vi "Validate Routing Channel.vi"(8 "error in (no error)":errorcluster, 11 "JSON RCT":refnum<class "JSON Routing Channel Template.lvclass">) -> (0 "error out":errorcluster, 3 "JSON RCT":refnum<class "JSON Routing Channel Template.lvclass">)   [LabVIEW 2020, in "Routing Templates.lvlib" / "JSON Routing Channel Template.lvclass"]
doc: "Throws error if the Routing Channel is not valid for any reason"
uses:
  JSON Routing Channel Template.lvclass
  JSON Routing Channel Template.lvclass/JSON Routing Channel Template.ctl
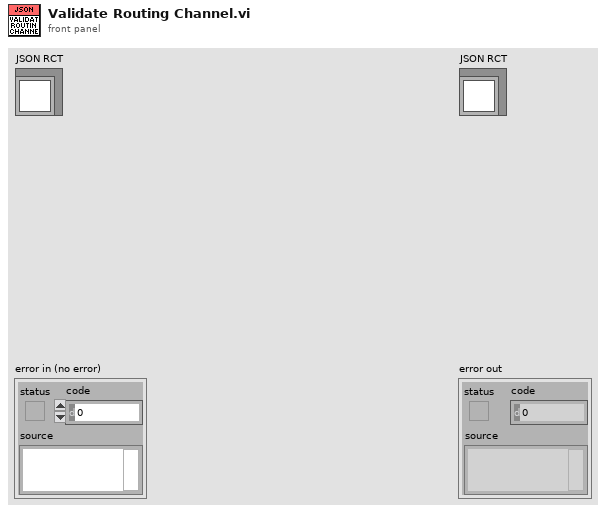
[diagram p1: front panel]
types:
  T1 = cluster{"Name":string, "Description":string, "Value":i32, "Connection List":cluster{"Channel":string, "Connection Type":string}[]}[]
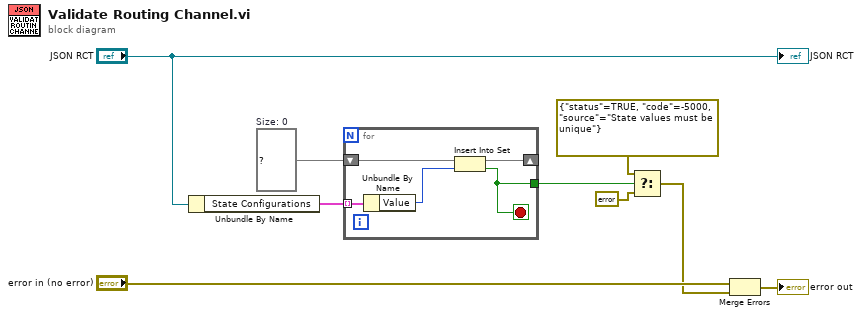
[diagram p0: block diagram]
diagram:
  w7 = set{i32} {}  # Size: 0
  n1 = Unbundle By Name("JSON RCT") -> ("State Configurations"=w8:T1)
  n2 = for {
    tunnel: w8 -> [w14] mode=indexing
    shift-right: [w11] -> _
    shift-left: w7 -> [w13]
    tunnel: [w10] -> w6
    stop <- w10 stop-if-true
    n3 = Unbundle By Name(w14) -> ("Value"=w12:i32)
    n4 = Insert Into Set(10:w12, 11:w13) -> (2:w10:bool, 3:w11:set{i32})
  }
  n5 = Select(t=errorcluster {"status"=TRUE, "code"=-5000, "source"="State values must be unique"} ("error constant"), s=w6, f=errorcluster {"status"=FALSE, "code"=0, "source"=""} ("error constant")) -> (s? t:f=w2:errorcluster)
  n6 = Merge Errors("error in (no error)", w2) -> (→"error out":errorcluster)
  "JSON RCT" <- "JSON RCT"
